vi "encodeStream.vi"(8 "error in (no error)":errorcluster, 11 "tBSONElement in":refnum<class "tBSONElement.lvclass">) -> (0 "error out":errorcluster, 2 "Byte Array":u8[](array[numeric]), 3 "tBSONElement out":refnum<class "tBSONElement.lvclass">)   [LabVIEW 2013, in "BSON.lvlib" / "tBSONElement.lvclass"]
doc: "Encodes a BSON element into a byte stream."
uses:
  tBSONElement.lvclass
  getName.vi
  BSON.lvlib
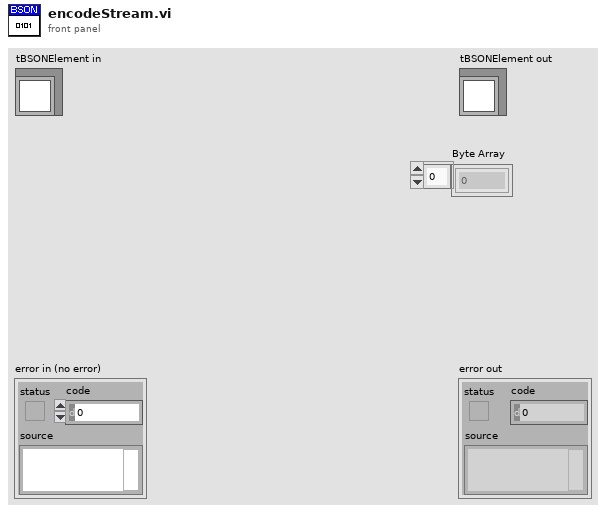
[diagram p1: front panel]
types:
  T1 = typedef "BSON.lvlib/tBSONElement.lvclass/type.ctl" = u8
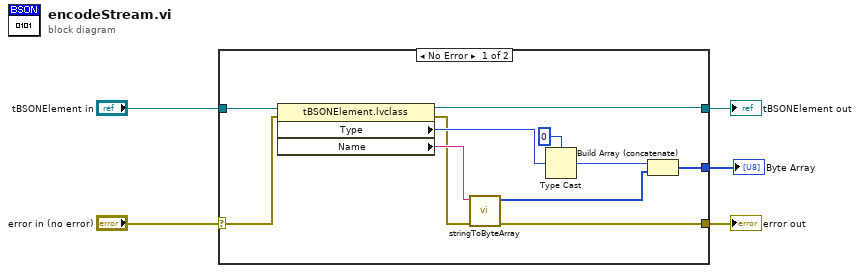
[diagram p0: block diagram]
diagram:
  n1 = case shown="No Error" "error in (no error)" {
    selector: "error in (no error)" -> [w15 w18]
    tunnel: [w6 w18] -> w4
    tunnel: [w12 w17] -> w2
    tunnel: "tBSONElement in" -> [w16 w17]
    tunnel: [w7 _] -> w1
    frame No Error {
      n2 = property class="tBSONElement.lvclass"(reference=w16, error in=w15) -> (reference out=w12:refnum<class "tBSONElement.lvclass">, error out=w10:errorcluster, "Type"=w13:T1, "Name"=w11:string)
      n3 = call "stringToByteArray.vi"("error in (no error)"=w10, "String"=w11) -> ("error out"=w6:errorcluster, "byte array"=w8:u8[])  [unwired: 8 in]
      n4 = Type Cast(type=u8 0, x=w13) -> (*(type *) &x=w9:u8)
      n5 = Build Array (concatenate)(w9, w8) -> (w7:u8[])
    }
    frame Error {
    }
  }
  "error out" <- w4
  "tBSONElement out" <- w2
  "Byte Array" <- w1
